vi "Autonomous.vi"() -> ()   [LabVIEW 2017]
doc: "This VI starts when autonomous period begins, and will automatically be terminated when it ends. You can carry out timed or sensor driven operations directly to I/O or to subsystems without needing to return to the caller."
uses:
  <vilib>/Rock Robotics/WPI/DriverStation/WPI_DriverStationPositionInfo.ctl
  <vilib>/Rock Robotics/Network Tables/NT Read String.vi
  Framework/Robot Global Data.vi
panel:
  in  "Switch Position":string
  in  "Robot Position":T1
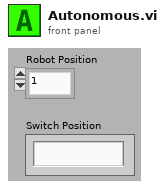
[diagram p1: front panel]
types:
  T1 = typedef "WPI_DriverStationPositionInfo.ctl" = enum16{"1", "2", "3"}
  T2 = cluster{"Auto Option":string, "Left Setpoint":dbl, "Right Setpoint":dbl, "Duration":dbl}[]
  T3 = typedef "Command Status Info.ctl" = cluster{"Name":string, "Status":T4, "notifier out":T5}
  T4 = typedef "Completion Status.ctl" = enum16{"Successful", "Aborted", "Incomplete"}
  T5 = typedef "Completion Notifier.ctl" = refnum<notifier>
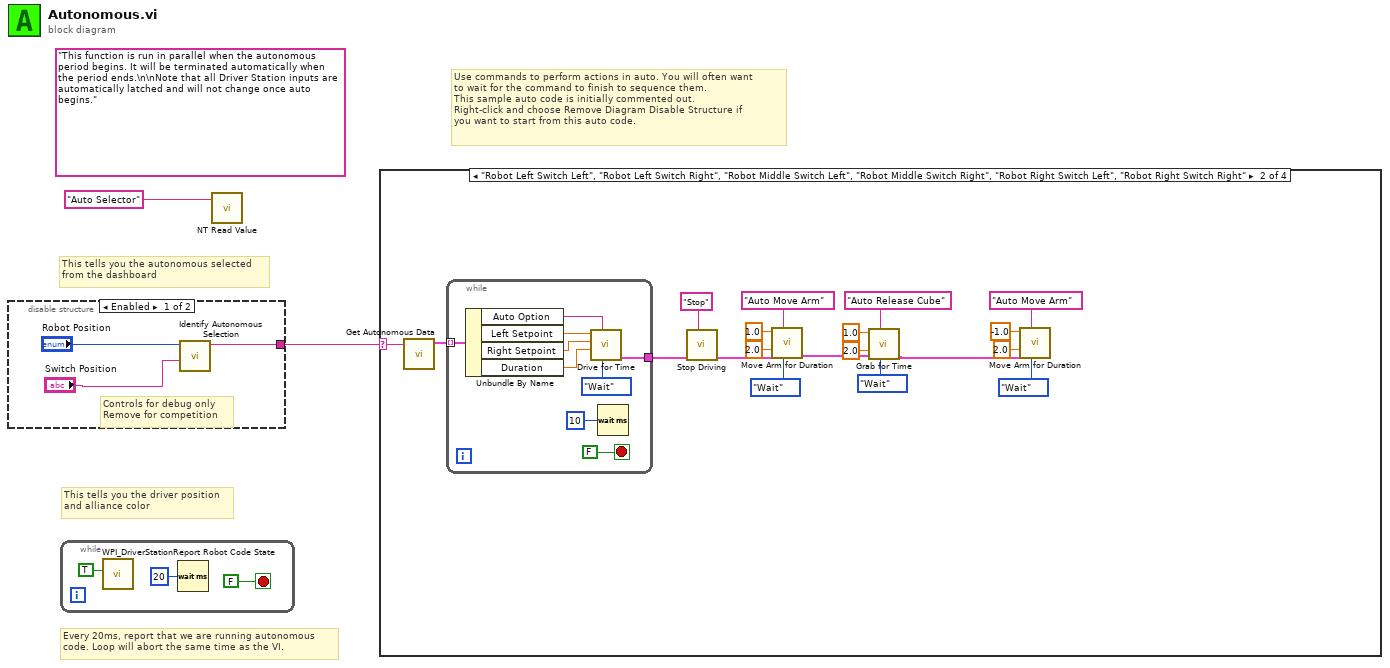
[diagram p0: block diagram]
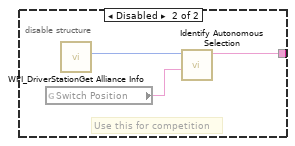
[diagram p2: hidden frame]
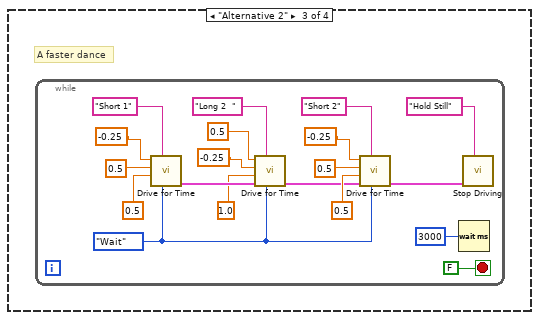
[diagram p4: hidden frame]
diagram:
  (unwired) "This function is run in parallel when the autonomous period begins. It will be terminated automatically when the period ends.\n\nNote that all Driver Station inputs are automatically latched and will not change once auto begins."
  # "This tells you the autonomous selected\nfrom the dashboard"
  # "Every 20ms, report that we are running autonomous\ncode. Loop will abort the same time as the VI."
  # "Use commands to perform actions in auto. You will often want\nto wait for the command to finish to sequence them.\nThis sample auto code is initially commented out. \nRight-click and choose Remove Diagram Disable Structure if\nyou want to start from this auto code."
  # "This tells you the driver position\nand alliance color"
  n1 = disable-structure shown="Enabled" {
    disable-tunnel: [w5 w6] -> w1
    frame Enabled {
      # "Controls for debug only\nRemove for competition"
      n2 = call "Identify Autonomous Selection.vi"("Switch Position"="Switch Position", "Robot Position"="Robot Position") -> ("Autonomous Selection"=w5:string)  [unwired: 9 in]
    }
    frame Disabled {
      # "Use this for competition"
      n3 = global read "Robot Global Data.vi" "Switch Position"() -> (w7:string)
      n4 = call <vilib>:"WPI_DriverStationGet Alliance Info.vi"() -> ("Position"=w8:T1)  [unwired: 11 out]
      n5 = call "Identify Autonomous Selection.vi"("Switch Position"=w7, "Robot Position"=w8) -> ("Autonomous Selection"=w6:string)  [unwired: 9 in]
    }
  }
  n6 = while {
    stop <- FALSE stop-if-true
    n7 = call <vilib>:"WPI_DriverStationReport Robot Code State.vi"("Autonomous"=TRUE) -> ()  [unwired: 10 in, 1 out]
    n8 = Wait (ms)(milliseconds to wait=u32 20) -> ()  [unwired: 1 out]
  }
  n9 = call-poly <vilib>:"NT Read Value.vi"("Name"="Auto Selector") -> ()  [unwired: 9 in, 2 out]
  n10 = case shown="\"Robot Left Switch Left\", \"Robot Left Switch Right\", \"Robot Middle Switch Left\", \"Robot Middle Switch Right\", \"Robot Right Switch Left\", \"Robot Right Switch Right\"" w1 {
    selector: w1 -> [_ w30 _ _]
    frame Default {
      # "You can put your main auto here, or you can right-click on the case and make any\nother frame be the default case."
      # "This is the frame that will execute if no selection is made, or if it is not recognized"
    }
    frame "Robot Left Switch Left", "Robot Left Switch Right", "Robot Middle Switch Left", "Robot Middle Switch Right", "Robot Right Switch Left", "Robot Right Switch Right" {
      n11 = call "Get Autonomous Data.vi"("Autonomous Selectin"=w30) -> ("Autonomous Data Selected"=w29:T2)  [unwired: 10 in]
      n12 = while {
        tunnel: w29 -> [w36] mode=indexing
        tunnel: [w31] -> w27
        stop <- FALSE stop-if-true
        n13 = Unbundle By Name(w36) -> ("Auto Option"=w35:string, "Left Setpoint"=w34:dbl, "Right Setpoint"=w33:dbl, "Duration"=w32:dbl)
        n14 = call "Drive for Time.vi"("Synchronization"=enum16{"Start", "Wait"}."Wait" ("Synchronication"), "Description"=w35, "Seconds"=w32, "Right Speed"=w33, "Left Speed"=w34) -> ("Command Info Out"=w31:T3)  [unwired: 5 in, 1 out]
        n15 = Wait (ms)(milliseconds to wait=u32 10 ("millisecond timer value")) -> ()  [unwired: 1 out]
      }
      n16 = call "Stop Driving.vi"("Description"="Stop", "Command Info In"=w27) -> ("Command Info Out"=w26:T3)  [unwired: 9 in]
      n17 = call "Move Arm for Duration.vi"("Synchronization"=enum16{"Start", "Wait"}."Wait", "Description"="Auto Move Arm", "Command Info In"=w26, "Duration (s)"=2.0, "Setpoint"=1.0) -> ("Command Info Out"=w21:T3)  [unwired: 6 in]
      n18 = call "Grab for Time.vi"("Synchronization"=enum16{"Start", "Wait"}."Wait", "Description"="Auto Release Cube", "Command Info In"=w21, "Duration (s)"=2.0, "Setpoint"=1.0) -> ("Command Info Out"=w12:T3)  [unwired: 6 in]
      n19 = call "Move Arm for Duration.vi"("Synchronization"=enum16{"Start", "Wait"}."Wait", "Description"="Auto Move Arm", "Command Info In"=w12, "Duration (s)"=2.0, "Setpoint"=-1.0) -> ()  [unwired: 6 in, 1 out]
    }
    frame "Alternative 2" {
      # "A faster dance"
      n20 = while {
        stop <- FALSE stop-if-true
        w40 = enum16{"Start", "Wait"}."Wait" ("Synchronication")
        n21 = call "Drive for Time.vi"("Synchronization"=w40, "Description"="Short 1", "Seconds"=0.5 ("Delay (s)"), "Right Speed"=0.5 ("X axis value"), "Left Speed"=-0.25 ("X axis value")) -> ("Command Info Out"=w58:T3)  [unwired: 5 in, 1 out]
        n22 = call "Drive for Time.vi"("Synchronization"=w40, "Description"="Long 2  ", "Command Info In"=w58, "Seconds"=1.0 ("Delay (s)"), "Right Speed"=-0.25 ("X axis value"), "Left Speed"=0.5 ("X axis value")) -> ("Command Info Out"=w42:T3)  [unwired: 4 in, 1 out]
        n23 = call "Drive for Time.vi"("Synchronization"=w40, "Description"="Short 2", "Command Info In"=w42, "Seconds"=0.5 ("Delay (s)"), "Right Speed"=0.5 ("X axis value"), "Left Speed"=-0.25 ("X axis value")) -> ("Command Info Out"=w41:T3)  [unwired: 4 in, 1 out]
        n24 = Wait (ms)(milliseconds to wait=u32 3000 ("millisecond timer value")) -> ()  [unwired: 1 out]
        n25 = call "Stop Driving.vi"("Description"="Hold Still", "Command Info In"=w41) -> ()  [unwired: 9 in, 1 out]
      }
    }
    frame "Your Turn" {
    }
  }
